vi "Icon Editor Init Refs.vi"(8 "error in":errorcluster, 10 "Ref Cluster":T1) -> (0 "error out":errorcluster)   [LabVIEW 2020]
uses:
  vi.lib/LabVIEW Icon API/lv_icon/Controls/Layer.ctl
  Controls/References Cluster.ctl
  lv_icon.lvlib
panel:
  in  "Localized tag":string="Import Icon from Owning Library"
  # "Localized Strings"
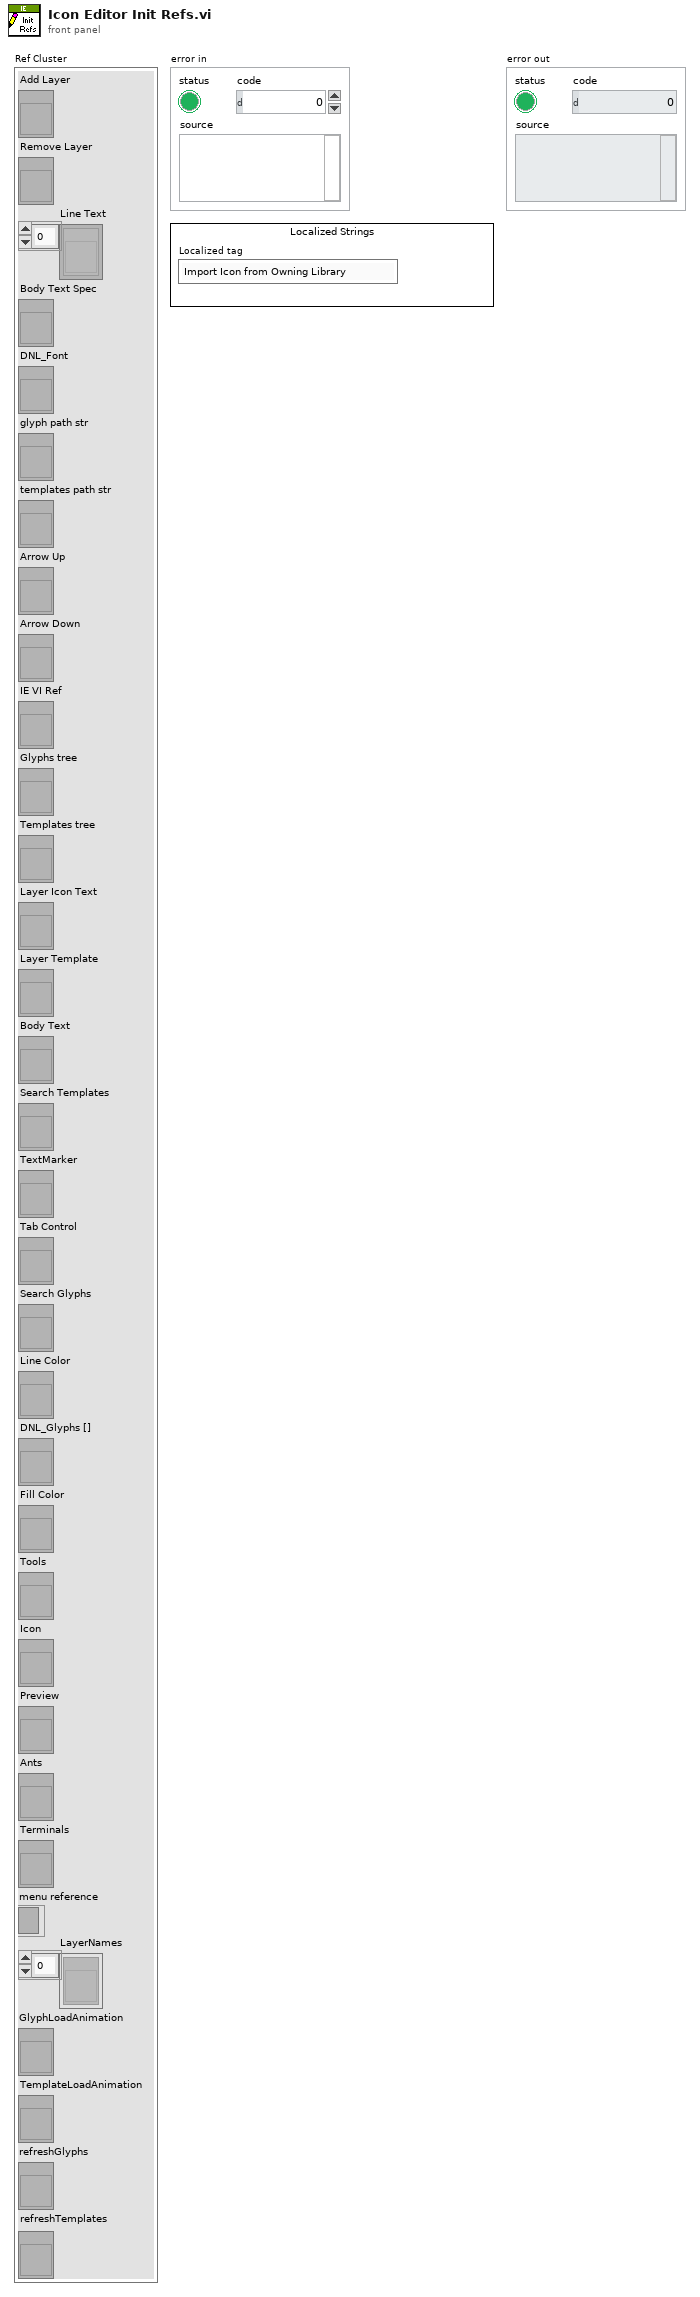
[diagram p1: front panel]
types:
  T1 = typedef "lv_icon.lvlib/References Cluster.ctl" = cluster{"Add Layer":refnum<vi>, "Remove Layer":refnum<vi>, "Line Text":refnum<vi>[], "Body Text Spec":refnum<vi>, "DNL_Font":refnum<vi>, "glyph path str":refnum<vi>, "templates path str":refnum<vi>, "Arrow Up":refnum<vi>, "Arrow Down":refnum<vi>, "IE VI Ref":refnum<vi>, "Glyphs tree":refnum<vi>, "Templates tree":refnum<vi>, "Layer Icon Text":refnum<vi>, "Layer Template":refnum<vi>, "Body Text":refnum<vi>, "Search Templates":refnum<vi>, "TextMarker":refnum<vi>, "Tab Control":refnum<vi>, "Search Glyphs":refnum<vi>, "Line Color":refnum<vi>, "DNL_Glyphs []":refnum<vi>, "Fill Color":refnum<vi>, "Tools":refnum<vi>, "Icon":refnum<vi>, "Preview":refnum<vi>, "Ants":refnum<vi>, "Terminals":refnum<vi>, "menu reference":refnum<k9>, "LayerNames":refnum<vi>[], "GlyphLoadAnimation":refnum<vi>, "TemplateLoadAnimation":refnum<vi>, "refreshGlyphs":refnum<vi>, "refreshTemplates":refnum<vi>}
  T2 = typedef "Layer.ctl" = cluster{"LayerIcon":picture, "LayerName":string, "Opacity":u8, "Visibility?":bool}
  T3 = enum8{"Enabled", "Disabled", "Disabled and Grayed Out"}
  T4 = typedef "lv_icon.lvlib/INI Data.ctl" = cluster{"Show Terminals?":bool, "Text":cluster{"Font":T5, "Alignment":T6, "Size":T7}, "3rd party Templates":cluster{"Store 3rd party Templates?":bool, "Folder Name":string}, "Merge user layers on commit":bool, "Body Text":T8, "Fill Color":T9, "Edge Color":T9, "Tab":u16, "Tool":T10, "Disable Layers?":bool}
  T5 = typedef "Font.ctl" = string
  T6 = typedef "Alignment.ctl" = u16
  T7 = typedef "Font Size.ctl" = u8
  T8 = typedef "BodyText.ctl" = cluster{"Line 1 text":string, "Line 2 text":string, "Line 3 text":string, "Line 4 text":string, "Line 1 color":u32, "Line 2 color":u32, "Line 3 color":u32, "Line 4 color":u32, "Body Text Spec":cluster{"Font":T5, "Alignment":T6, "Size":u8}, "Center text vertically":bool, "Capitalize Text":bool}
  T9 = typedef "IEColor.ctl" = u32
  T10 = typedef "Tools.ctl" = enum32{"Pencil", "Line", "Dropper", "Fill", "Rectangle", "Filled Rectangle", "Ellipse", "Filled Ellipse", "Eraser", "Text", "Select", "Move"}
  T11 = typedef "LabVIEW Icon Stored Information.ctl" = cluster{"Text Visible?":bool, "Text Opacity":u8, "Templ Visible?":bool, "Templ Opacity":u8, "Relative Path from 1 to 2":path, "Image":picture, "All User Layers":refnum<class "Layer.lvclass">[], "Body Text":T8}
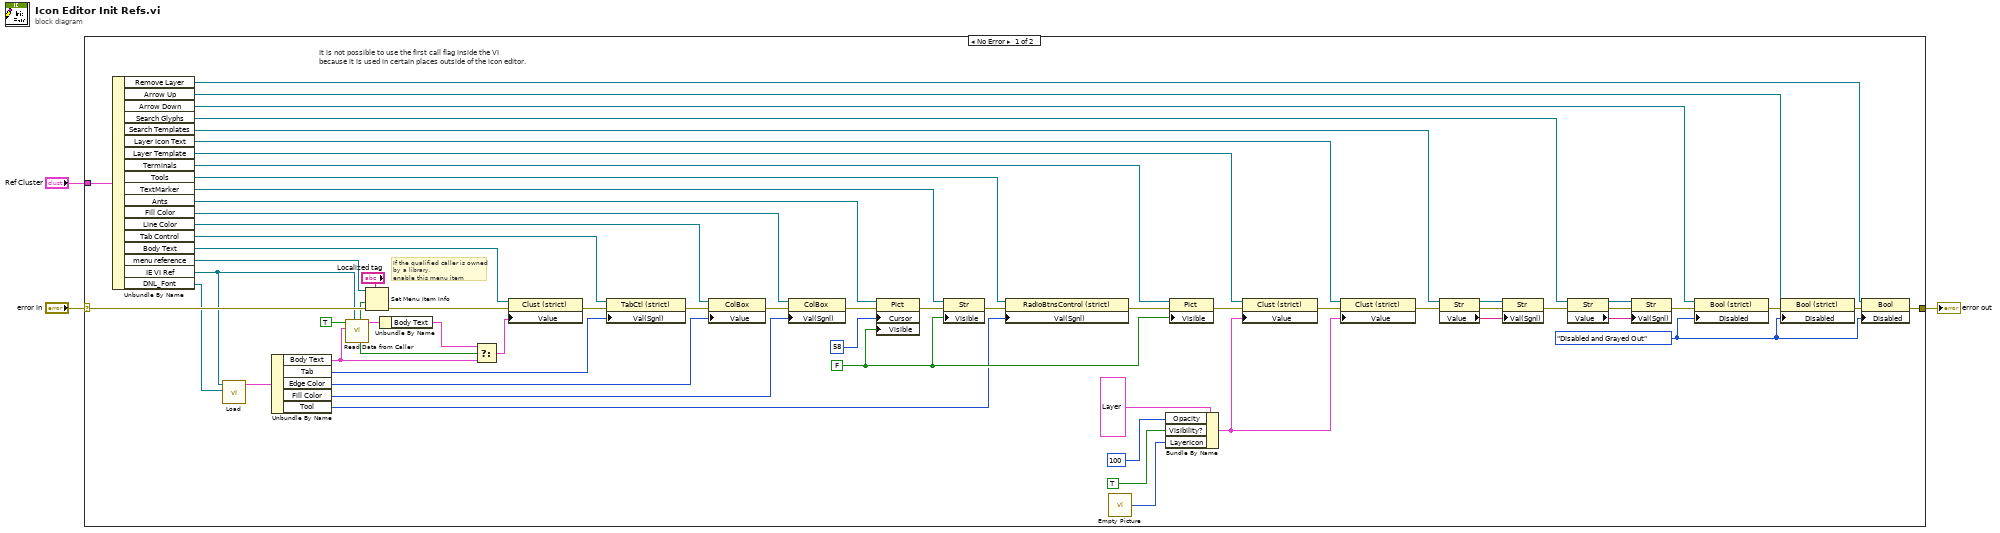
[diagram p0: block diagram]
diagram:
  n1 = case shown="No Error" "error in" {
    selector: "error in" -> [w49 w67]
    tunnel: [w50 w67] -> w2
    tunnel: "Ref Cluster" -> [w31 _]
    frame No Error {
      w4 = T3."Disabled and Grayed Out" ("Disabled")
      w36 = FALSE ("Visible")
      # "If the qualified caller is owned by a library,\nenable this menu item"
      # "It is not possible to use the first call flag inside the VI\nbecause it is used in certain places outside of the icon editor."
      n2 = Unbundle By Name(w31) -> ("Remove Layer"=w16:refnum<vi>, "Arrow Up"=w29:refnum<vi>, "Arrow Down"=w30:refnum<vi>, "Search Glyphs"=w23:refnum<vi>, "Search Templates"=w28:refnum<vi>, "Layer Icon Text"=w19:refnum<vi>, "Layer Template"=w32:refnum<vi>, "Terminals"=w37:refnum<vi>, "Tools"=w38:refnum<vi>, "TextMarker"=w39:refnum<vi>, "Ants"=w41:refnum<vi>, "Fill Color"=w46:refnum<vi>, "Line Color"=w47:refnum<vi>, "Tab Control"=w35:refnum<vi>, "Body Text"=w17:refnum<vi>, "menu reference"=w13:refnum<k9>, "IE VI Ref"=w10:refnum<vi>, "DNL_Font"=w9:refnum<vi>)
      n3 = call "Load.vi"("DNL_Font"=w9, "IE VI Ref"=w10) -> ("INI Data"=w12:T4)  [unwired: 1 in, 8 out]
      n4 = Unbundle By Name(w12) -> ("Body Text"=w11:T8, "Tab"=w8:u16, "Edge Color"=w7:T9, "Fill Color"=w6:T9, "Tool"=w5:T10)
      n5 = call "Read Data from Caller.vi"("lv_icon.vi"=w10, "Default body text"=w11, "Init? (F)"=TRUE) -> ("data"=w44:T11, "Valid?"=w45:bool, "Valid Library icon?"=w14:bool)  [unwired: 1 in, 5 out]
      n6 = Set Menu Item Info(7:"Localized tag", 8:w49, 9:w14, 11:w13) -> (0:w48:errorcluster)  [unwired: 3 in, 1 out]
      n7 = Unbundle By Name(w44) -> ("Body Text"=w43:T8)
      n8 = Select(t=w43, s=w45, f=w11) -> (s? t:f=w42:T8)
      n9 = property class="Clust (strict)"(reference=w17, error in=w48, "Value"=w42) -> (error out=w53:errorcluster)  [unwired: 1 out]
      n10 = property class="TabCtl (strict)"(reference=w35, error in=w53, "Val(Sgnl)"=w8) -> (error out=w62:errorcluster)  [unwired: 1 out]
      n11 = property class="ColBox"(reference=w47, error in=w62, "Value"=w7) -> (error out=w66:errorcluster)  [unwired: 1 out]
      n12 = property class="ColBox"(reference=w46, error in=w66, "Val(Sgnl)"=w6) -> (error out=w52:errorcluster)  [unwired: 1 out]
      n13 = property class="Pict"(reference=w41, error in=w52, "Cursor"=58, "Visible"=w36) -> (error out=w65:errorcluster)  [unwired: 1 out]
      n14 = property class="Str"(reference=w39, error in=w65, "Visible"=w36) -> (error out=w64:errorcluster)  [unwired: 1 out]
      n15 = property class="RadioBtnsControl (strict)"(reference=w38, error in=w64, "Val(Sgnl)"=w5) -> (error out=w63:errorcluster)  [unwired: 1 out]
      n16 = call "Empty Picture"() -> ("empty picture"=w33:picture)
      n17 = Bundle By Name(cluster=T2 {"LayerIcon"=bytes[0], "LayerName"="", "Opacity"=0, "Visibility?"=FALSE} ("Value (Signaling)"), "Opacity"=u8 100, "Visibility?"=TRUE, "LayerIcon"=w33) -> (w18:T2)
      n18 = property class="Pict"(reference=w37, error in=w63, "Visible"=w36) -> (error out=w61:errorcluster)  [unwired: 1 out]
      n19 = property class="Clust (strict)"(reference=w32, error in=w61, "Value"=w18) -> (error out=w55:errorcluster)  [unwired: 1 out]
      n20 = property class="Clust (strict)"(reference=w19, error in=w55, "Value"=w18) -> (error out=w54:errorcluster)  [unwired: 1 out]
      n21 = property class="Str"(reference=w28, error in=w54) -> (reference out=w27:refnum<vi>, error out=w59:errorcluster, "Value"=w26:string)
      n22 = property class="Str"(reference=w27, error in=w59, "Val(Sgnl)"=w26) -> (error out=w57:errorcluster)  [unwired: 1 out]
      n23 = property class="Str"(reference=w23, error in=w57) -> (reference out=w24:refnum<vi>, error out=w58:errorcluster, "Value"=w25:string)
      n24 = property class="Str"(reference=w24, error in=w58, "Val(Sgnl)"=w25) -> (error out=w56:errorcluster)  [unwired: 1 out]
      n25 = property class="Bool (strict)"(reference=w30, error in=w56, "Disabled"=w4) -> (error out=w60:errorcluster)  [unwired: 1 out]
      n26 = property class="Bool (strict)"(reference=w29, error in=w60, "Disabled"=w4) -> (error out=w51:errorcluster)  [unwired: 1 out]
      n27 = property class="Bool"(reference=w16, error in=w51, "Disabled"=w4) -> (error out=w50:errorcluster)  [unwired: 1 out]
    }
    frame Error {
    }
  }
  "error out" <- w2
